vi "Conversions.vi"() -> ()   [LabVIEW 2011]
panel:
  out "element":bool
  out "Boolean array":bool[](array[boolean])
  in  "Enum":enum16{"OFF", "ON"}(ring)
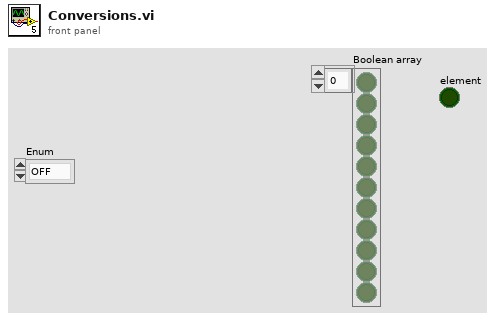
[diagram p1: front panel]
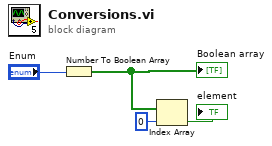
[diagram p0: block diagram]
diagram:
  n1 = Number To Boolean Array(number="Enum") -> (Boolean array=w3:bool[])
  "Boolean array" <- w3
  n2 = Index Array(array=w3, index=0) -> (element=→"element":bool)
